vi "loopprpoerties2.vi"() -> ()   [LabVIEW 2019]
panel:
  out "x = y?":bool[](array[boolean])
  out "Array 4":dbl[](array[numeric])
  out "Waveform Graph":dbl[](graph)
  in  "Numeric 4":dbl
  out "Numeric 3":i16
  in  "stop":bool
  in  "String 3":string
  in  "String 2":string
  out "Numeric 2":i8
  out "Array 3":i8[](array[numeric])
  out "String":string
  out "Array 2":dbl[](array[numeric])
  out "Array":dbl[][](array[numeric])
  in  "Numeric":dbl
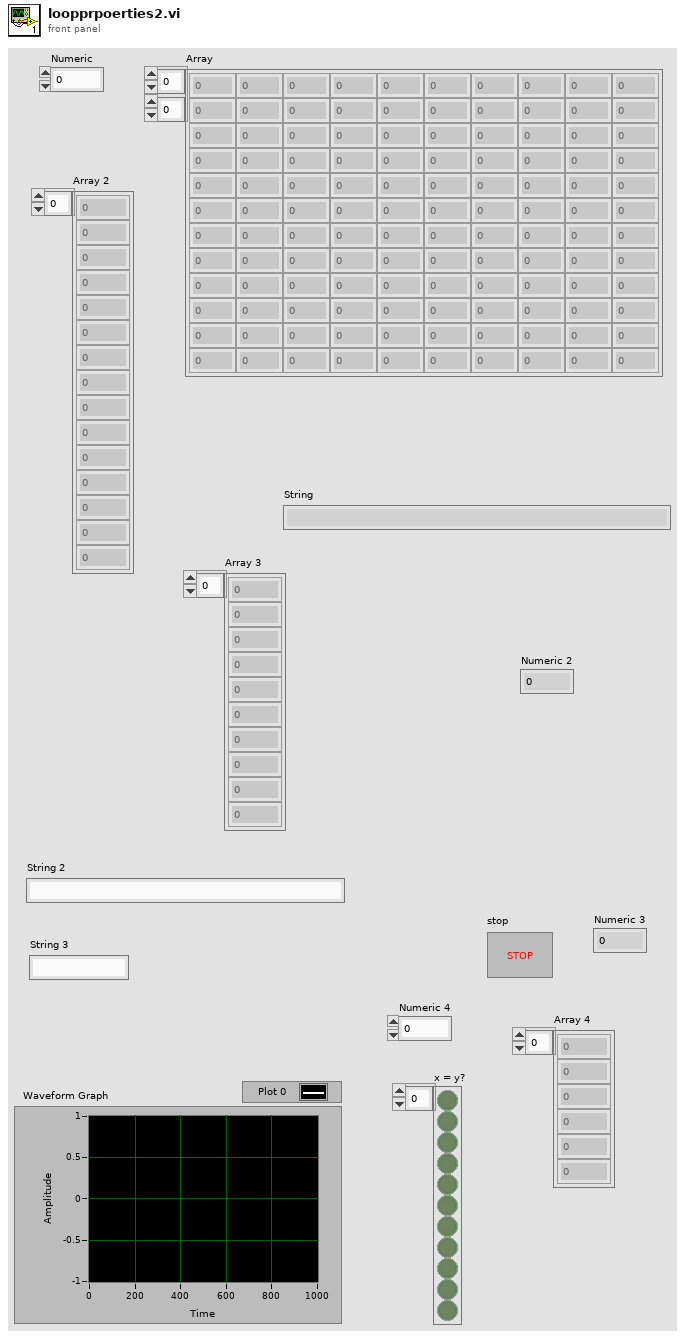
[diagram p1: front panel]
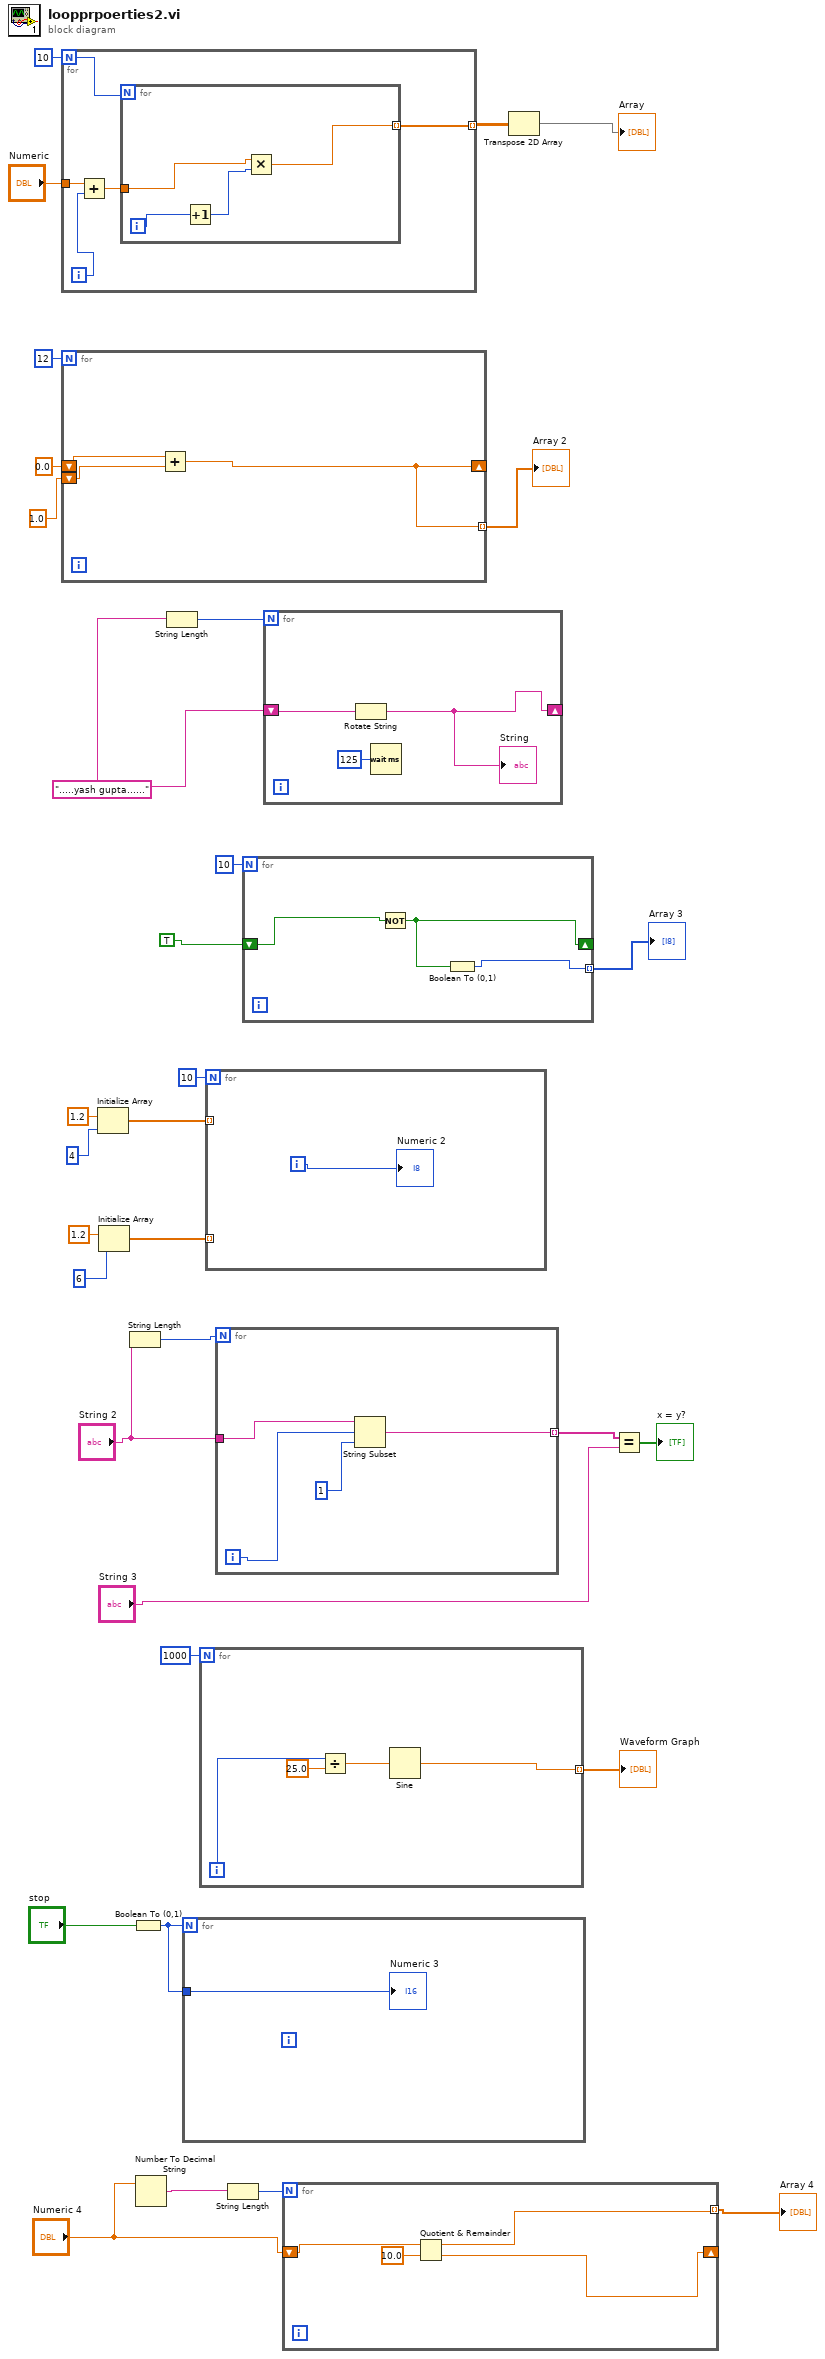
[diagram p0: block diagram]
diagram:
  w26 = ".....yash gupta......"
  n1 = for {
    N: 10 -> [w38]
    tunnel: "Numeric" -> [w35]
    tunnel: [w34] -> w6 mode=indexing
    i -> [w36]
    n2 = Add(x=w35, y=w36) -> (x+y=w37:dbl)
    n3 = for {
      N: w38 -> [_]
      tunnel: w37 -> [w40]
      tunnel: [w39] -> w34 mode=indexing
      i -> [w42]
      n4 = Increment(x=w42) -> (x+1=w41:i32)
      n5 = Multiply(x=w40, y=w41) -> (x*y=w39:dbl)
    }
  }
  n6 = for {
    N: 12 -> [_]
    shift-right: [w43] -> _
    shift-left: 0.0 -> [w45]
    shift-left: 1.0 -> [w44]
    tunnel: [w43] -> w28 mode=indexing
    n7 = Add(x=w45, y=w44) -> (x+y=w43:dbl)
  }
  "Array 2" <- w28
  n8 = Initialize Array "Initialize Array"(1.2 ("element"), 4 ("dimension size")) -> (w17:dbl[])
  n9 = Initialize Array(1.2 ("element"), 6 ("dimension size")) -> (w16:dbl[])
  n10 = String Length(string="String 2") -> (length=w15:i32)
  n11 = Boolean To (0,1)(Boolean="stop") -> (0, 1=w3:i16)
  n12 = Number To Decimal String(number="Numeric 4") -> (decimal integer string=w8:string)  [unwired: 1 in]
  n13 = String Length(string=w26) -> (length=w27:i32)
  n14 = for {
    N: w3 -> [_]
    tunnel: w3 -> [w46]
    "Numeric 3" <- w46
  }
  n15 = for {
    N: 1000 -> [_]
    tunnel: [w47] -> w4 mode=indexing
    i -> [w49]
    n16 = Divide(x=w49, y=25.0) -> (x/y=w48:dbl)
    n17 = Sine(x=w48) -> (sin(x)=w47:dbl)
  }
  "Waveform Graph" <- w4
  n18 = for {
    N: 10 -> [_]
    tunnel: w17 -> [_] mode=indexing
    tunnel: w16 -> [_] mode=indexing
    i -> [w51]
    "Numeric 2" <- w51
  }
  n19 = for {
    N: w15 -> [_]
    tunnel: "String 2" -> [w55]
    tunnel: [w52] -> w13 mode=indexing
    i -> [w54]
    n20 = String Subset(string=w55, offset (0)=w54, length (rest)=1 ("length (rest)")) -> (substring=w52:string)
  }
  n21 = String Length(string=w8) -> (length=w9:i32)
  n22 = for {
    N: 10 -> [_]
    shift-right: [w57] -> _
    shift-left: TRUE -> [w58]
    tunnel: [w56] -> w23 mode=indexing
    n23 = Not(x=w58) -> (.not. x?=w57:bool)
    n24 = Boolean To (0,1)(Boolean=w57) -> (0, 1=w56:i16)
  }
  "Array 3" <- w23
  n25 = for {
    N: w27 -> [_]
    shift-right: [w60] -> _
    shift-left: w26 -> [w61]
    n26 = Rotate String(1:w61) -> (0:w60:string)
    "String" <- w60
    n27 = Wait (ms)(milliseconds to wait=u32 125) -> ()  [unwired: 1 out]
  }
  n28 = for {
    N: w9 -> [_]
    shift-right: [w63] -> _
    shift-left: "Numeric 4" -> [w65]
    tunnel: [w62] -> w2 mode=indexing
    n29 = Quotient & Remainder(x=w65, y=10.0) -> (x-y*floor(x/y)=w62:dbl, floor(x/y)=w63:dbl)
  }
  "Array 4" <- w2
  n30 = Transpose 2D Array(2D array=w6) -> (transposed array=→"Array":dbl[][])
  n31 = Equal?(x=w13, y="String 3") -> (x = y?=→"x = y?":bool[])
